vi "Heat Up Macro HEWH Type.vi"(8 "Error In":errorcluster, 11 "Heat Up Data with Only Selected Columns":string[][](array[string])) -> (0 "Error Out":errorcluster, 2 "Gallon Target":dbl, 3 "Water Heater Type":T1)   [LabVIEW 2016]
uses:
  Type Definitions/HEWH_Type.ctl
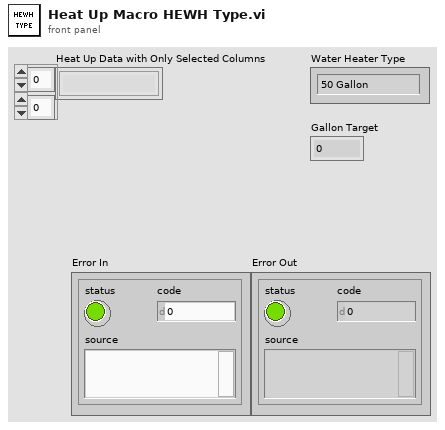
[diagram p1: front panel]
types:
  T1 = typedef "HEWH_Type.ctl" = enum16{"50 Gallon", "80 Gallon"}
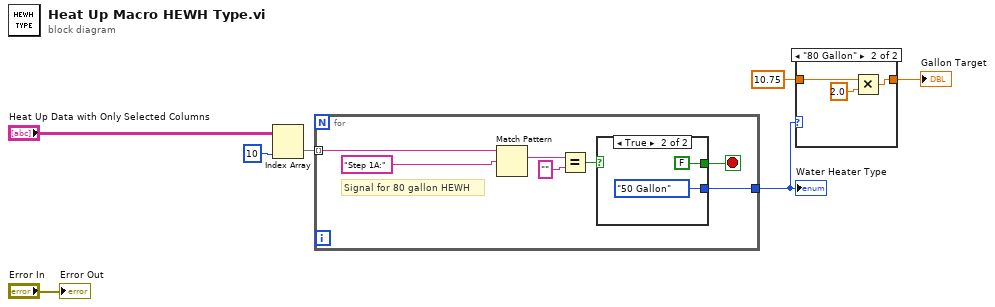
[diagram p0: block diagram]
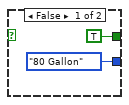
[diagram p2: hidden frame]
diagram:
  n1 = Index Array(array="Heat Up Data with Only Selected Columns", index (col)=10 ("disabled index (col)")) -> (element=w5:string[])  [unwired: 1 in]
  n2 = for {
    tunnel: w5 -> [w14] mode=indexing
    tunnel: [w9] -> w6
    stop <- w10 stop-if-true
    # "Signal for 80 gallon HEWH"
    n3 = Match Pattern(string=w14, regular expression="Step 1A:") -> (match substring=w8:string)  [unwired: 1 in, 3 out]
    n4 = Equal?(x=w8, y="") -> (x = y?=w11:bool)
    n5 = case shown="True" w11 {
      tunnel: [TRUE FALSE] -> w10
      tunnel: [HEWH_Type."80 Gallon" ("Water Heater Type") HEWH_Type."50 Gallon" ("Water Heater Type")] -> w9
      frame False {
      }
      frame True {
      }
    }
  }
  "Water Heater Type" <- w6
  n6 = case shown="\"80 Gallon\"" w6 {
    tunnel: [w19 w22] -> w2
    tunnel: 10.75 ("y") -> [w19 w21]
    frame "50 Gallon", Default {
    }
    frame "80 Gallon" {
      n7 = Multiply(x=w21, y=2.0) -> (x*y=w22:dbl)
    }
  }
  "Gallon Target" <- w2
  "Error Out" <- "Error In"
